vi "_getNextToken.vi"(8 "error in (no error)":errorcluster, 11 "JSON Parser In":refnum<class "tJSONParser.lvclass">) -> (0 "error out":errorcluster, 3 "JSON Parser Out":refnum<class "tJSONParser.lvclass">)   [LabVIEW 2013, in "JSON.lvlib" / "tJSONParser.lvclass"]
doc: "Removes all whitespace and comments from the JSON string up to and including the first valid JSON token. The line number is incremented each time a newline is encountered. The type of the JSON token is set on the tJasonParser object."
uses:
  tJSONParser.lvclass
  tJSONParser.lvclass/tJSONParser.ctl
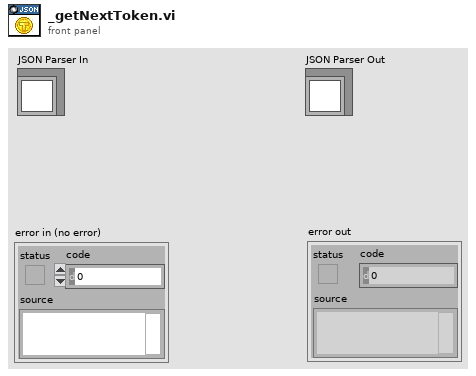
[diagram p1: front panel]
types:
  T1 = typedef "JSON.lvlib/tJSONParser.lvclass/_tokenType.ctl" = enum16{"Object Begin", "Object End", "Array Begin", "Array End", "String Delimeter", "Forward Slash", "Number", "Boolean", "Null", "Object Or Array Separator", "Pair Separator", "End Of File", "Asterisk", "Backward Slash", "Other"}
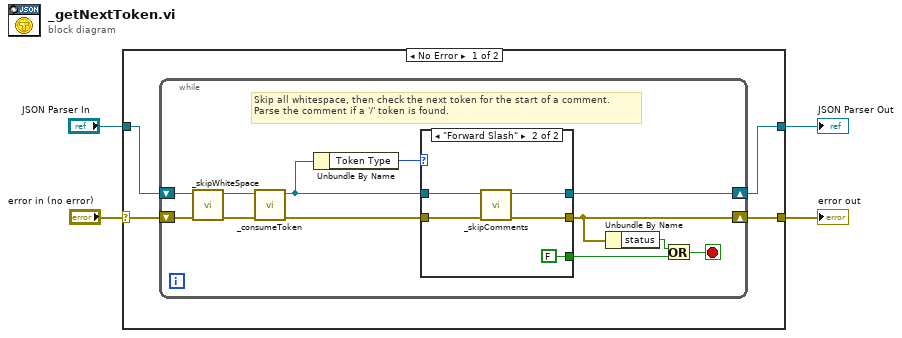
[diagram p0: block diagram]
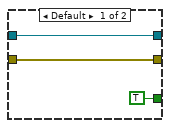
[diagram p2: hidden frame]
diagram:
  n1 = case shown="No Error" "error in (no error)" {
    selector: "error in (no error)" -> [w8 w30]
    tunnel: [w6 w30] -> w3
    tunnel: "JSON Parser In" -> [w7 w29]
    tunnel: [w5 w29] -> w1
    frame No Error {
      n2 = while {
        shift-right: [w11] -> w5
        shift-left: w7 -> [w19]
        shift-right: [w15] -> w6
        shift-left: w8 -> [w20]
        stop <- w14 stop-if-true
        # "Skip all whitespace, then check the next token for the start of a comment.\nParse the comment if a '/' token is found."
        n3 = call "_skipWhiteSpace.vi"("error in (no error)"=w20, "JSON Parser In"=w19) -> ("error out"=w17:errorcluster, "JSON Parser Out"=w18:refnum<class "tJSONParser.lvclass">)  [unwired: 5 in, 3 out]
        n4 = call "_consumeToken.vi"("error in (no error)"=w17, "JSON Parser In"=w18) -> ("error out"=w16:errorcluster, "JSON Parser Out"=w10:refnum<class "tJSONParser.lvclass">)  [unwired: 8 in]
        n5 = Unbundle By Name(w10) -> ("Token Type"=w9:T1)
        n6 = case shown="\"Forward Slash\"" w9 {
          tunnel: w10 -> [w23 w26]
          tunnel: w16 -> [w22 w27]
          tunnel: [w22 w24] -> w15
          tunnel: [TRUE FALSE] -> w12
          tunnel: [w23 w25] -> w11
          frame Default {
          }
          frame "Forward Slash" {
            n7 = call "_skipComments.vi"("error in (no error)"=w27, "JSON Parser In"=w26) -> ("error out"=w24:errorcluster, "JSON Parser Out"=w25:refnum<class "tJSONParser.lvclass">)  [unwired: 8 in]
          }
        }
        n8 = Unbundle By Name(w15) -> ("status"=w13:bool)
        n9 = Or(x=w13, y=w12) -> (x .or. y?=w14:bool)
      }
    }
    frame Error {
    }
  }
  "error out" <- w3
  "JSON Parser Out" <- w1
